vi "ConvValid.vi"(11 "Path":path) -> (3 "Valid":bool)   [LabVIEW 2022 SP3]
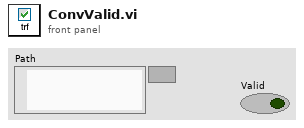
[diagram p1: front panel]
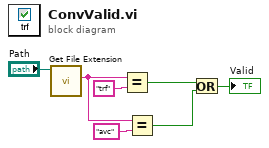
[diagram p0: block diagram]
diagram:
  n1 = call <vilib>:"Get File Extension.vi"("file"="Path") -> ("lowercase file extension"=w3:string)  [unwired: 6 in, 4 out]
  n2 = Equal?(x=w3, y="trf" ("element")) -> (x = y?=w5:bool)
  n3 = Equal?(x=w3, y="avc" ("element")) -> (x = y?=w6:bool)
  n4 = Or(x=w5, y=w6) -> (x .or. y?=→"Valid":bool)
